vi "Example.vi"() -> ()   [LabVIEW 2013]
uses:
  ToolbarMenu/MenuPosition.ctl
  ToolbarMenu/ToolbarMenu.lvlib
panel:
  in  "Hamburger Menu Button":bool
  in  "Menu Button":bool
  in  "Exit on VI Deactivation (T)":bool=TRUE
  in  "ExitControls (Empty for all)":string[](array[string])
  out "ExitControl":cluster{"Name":string, "Value":variant}
  in  "Dim Transparency":u8=80
  in  "DimRegion":enum16{"VI", "Control", "Screen"}(ring)
  in  "MenuPosition":T1=enum."BottomToRight"
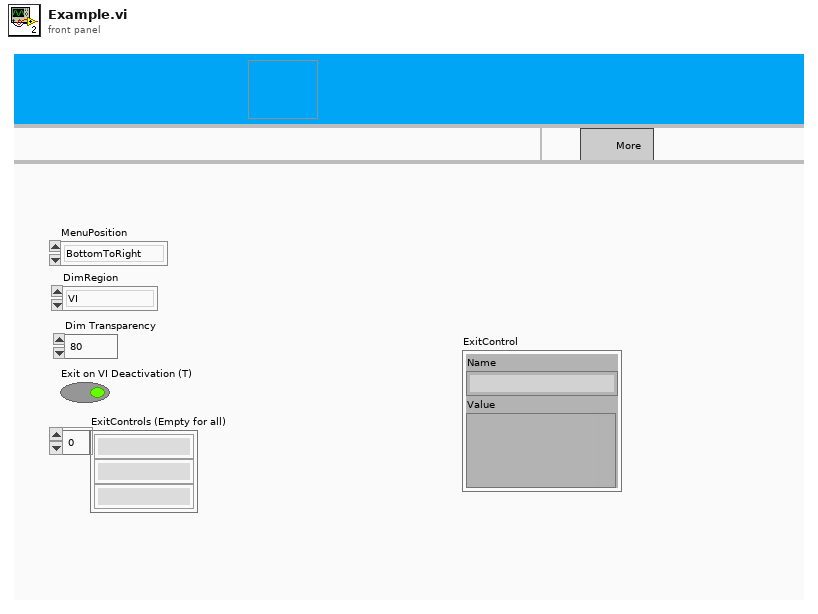
[diagram p1: front panel]
types:
  T1 = typedef "ToolbarMenu.lvlib/MenuPosition.ctl" = enum16{"TopToRight", "BottomToRight", "TopToLeft", "BottomToLeft"}
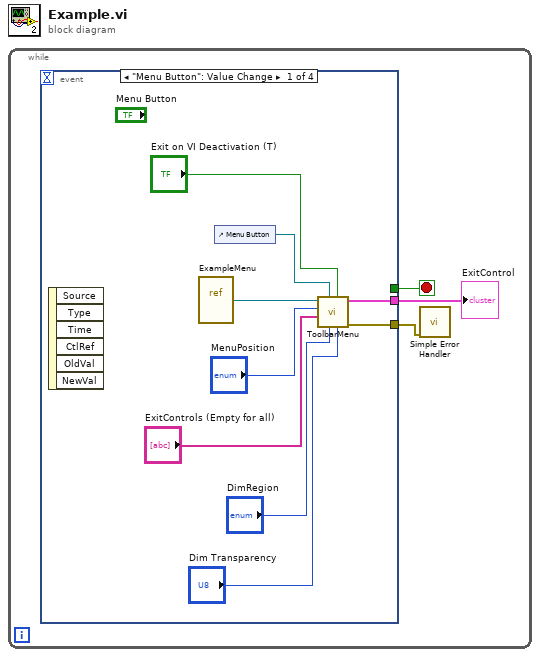
[diagram p0: block diagram]
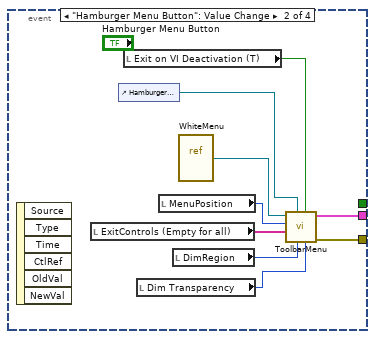
[diagram p2: hidden frame]
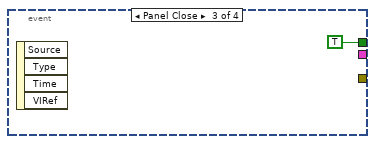
[diagram p3: hidden frame]
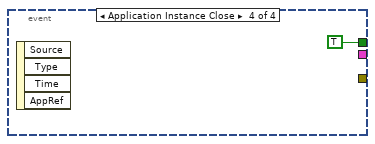
[diagram p4: hidden frame]
diagram:
  n1 = while {
    stop <- w3 stop-if-true
    n2 = event shown="[0] \"Menu Button\": Value Change" {
      selector: _ -> [_ _ _ _]
      dyn-events: _ -> [_ _ _ _]
      timeout: _ -> [_ _ _ _]
      tunnel: [_ _ TRUE TRUE] -> w3
      tunnel: [w10 w21 _ _] -> w2
      tunnel: [w9 w18 _ _] -> w1
      event "Menu Button": Value Change {
        n3 = event-data() -> ()  [unwired: 1 in, 6 out]
        n4 = vi-ref "ExampleMenu.vi"() -> (w12:refnum<vi>)
        n5 = control-ref of="Menu Button"() -> (w11:refnum<vi>)
        n6 = call "ToolbarMenu.vi"("Dim Transparency (90)"="Dim Transparency", "Exit on VI Deactivation (T)"="Exit on VI Deactivation (T)", "DimRegion (VI)"="DimRegion", "Caller Control Refnum"=w11, "ExitControls (Empty for all)"="ExitControls (Empty for all)", "Position"="MenuPosition", "Menu Vi Reference"=w12) -> ("error out"=w9:errorcluster, "ExitControl"=w10:cluster{"Name":string, "Value":variant})  [unwired: 3 in]
      }
      event "Hamburger Menu Button": Value Change {
        n7 = event-data() -> ()  [unwired: 1 in, 6 out]
        n8 = local read "ExitControls (Empty for all)"() -> (w16:string[])
        n9 = control-ref of="Hamburger Menu Button"() -> (w20:refnum<vi>)
        n10 = local read "Exit on VI Deactivation (T)"() -> (w13:bool)
        n11 = local read "Dim Transparency"() -> (w14:u8)
        n12 = local read "MenuPosition"() -> (w17:T1)
        n13 = local read "DimRegion"() -> (w15:enum16{"VI", "Control", "Screen"})
        n14 = vi-ref "WhiteMenu.vi"() -> (w19:refnum<vi>)
        n15 = call "ToolbarMenu.vi"("Dim Transparency (90)"=w14, "Exit on VI Deactivation (T)"=w13, "DimRegion (VI)"=w15, "Caller Control Refnum"=w20, "ExitControls (Empty for all)"=w16, "Position"=w17, "Menu Vi Reference"=w19) -> ("error out"=w18:errorcluster, "ExitControl"=w21:cluster{"Name":string, "Value":variant})  [unwired: 3 in]
      }
      event Panel Close {
        n16 = event-data() -> ()  [unwired: 1 in, 4 out]
      }
      event Application Instance Close {
        n17 = event-data() -> ()  [unwired: 1 in, 4 out]
      }
    }
    "ExitControl" <- w2
    n18 = call <vilib>:"Simple Error Handler.vi"("error in (no error)"=w1) -> ()  [unwired: 4 in, 5 out]
  }
